vi "Set Current Velocity Period.vi"(8 "error in (no error)":errorcluster, 10 "period (0: off)":u16, 11 "DC Brick in":refnum<class "DC Brick.lvclass">) -> (0 "error out":errorcluster, 3 "DC Brick out":refnum<class "DC Brick.lvclass">)   [LabVIEW 2011, in "Tinkerforge.lvlib" / "DC Brick.lvclass"]
doc: "This VI sets a period in ms with which the CALLBACK_CURRENT_VELOCITY callback is triggered. A period of 0 turns the callback off.\n\nThe default value is 0."
uses:
  DC Brick.lvclass
  Device/Device.lvclass
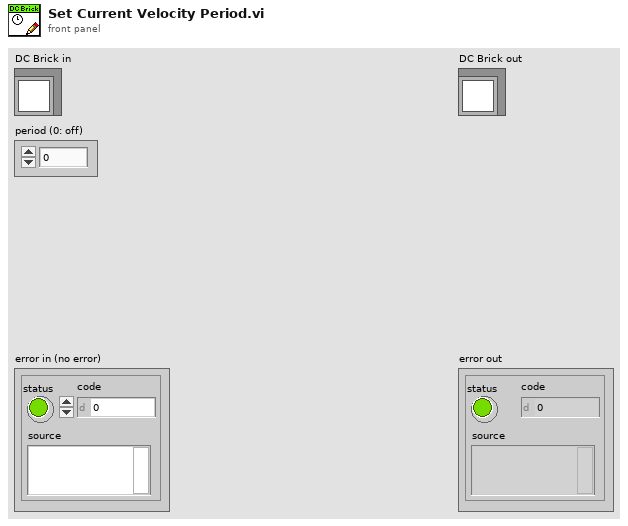
[diagram p1: front panel]
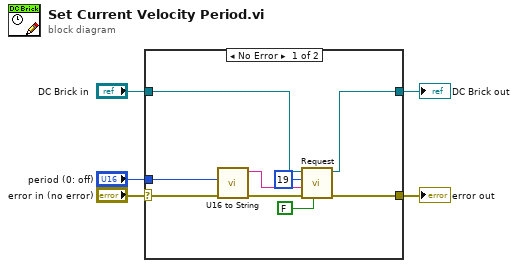
[diagram p0: block diagram]
diagram:
  n1 = case shown="No Error" "error in (no error)" {
    selector: "error in (no error)" -> [w9 w16]
    tunnel: [w10 w16] -> w4
    tunnel: [w13 w15] -> w2
    tunnel: "DC Brick in" -> [w14 w15]
    tunnel: "period (0: off)" -> [w7 _]
    frame No Error {
      n2 = call "U16 to String.vi"("Error In"=w9, "U16"=w7) -> ("Error Out"=w8:errorcluster, "String out"=w6:string)  [unwired: 8 in]
      n3 = call "Request.vi"("Response"=FALSE, "error in (no error)"=w8, "Data"=w6, "Function ID"=u8 19, "Device in"=w14) -> ("error out"=w10:errorcluster, "Device out"=w13:refnum<class "DC Brick.lvclass">)  [unwired: 2 in, 3 out]
    }
    frame Error {
    }
  }
  "error out" <- w4
  "DC Brick out" <- w2
